vi "Tx_ack.vi"(3 "error in (no error)":errorcluster, 4 "txbuf":string, 5 "VISA resource name":refnum<visa-resource-name>="COM255") -> (0 "error out":errorcluster, 1 "envio OK":bool, 2 "VISA resource name OUT":refnum<visa-resource-name>)   [LabVIEW 2018]
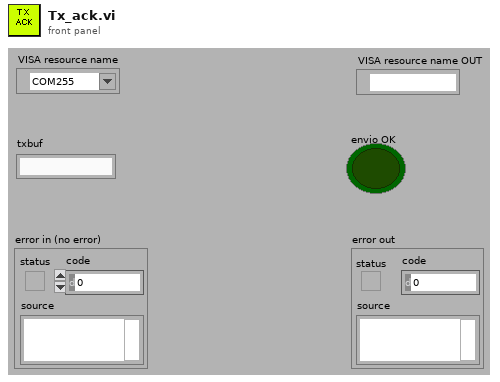
[diagram p1: front panel]
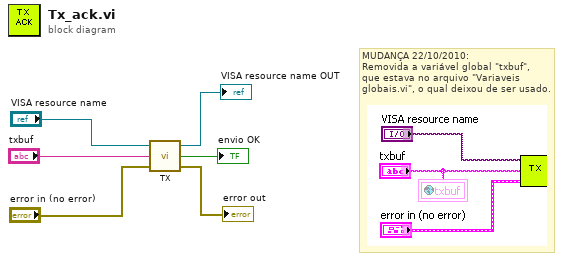
[diagram p0: block diagram]
diagram:
  # "MUDANÇA 22/10/2010:\nRemovida a variável global \"txbuf\",\nque estava no arquivo \"Variaveis globais.vi\", o qual deixou de ser usado."
  n1 = call "TX.vi"("error in (no error)"="error in (no error)", "tx_buf"="txbuf", "VISA resource name"="VISA resource name") -> ("error out"=→"error out":errorcluster, "envio OK"=→"envio OK":bool, "VISA resource name OUT"=→"VISA resource name OUT":refnum<visa-resource-name>)
